vi "Apply Transfer Function.vi"() -> ()   [LabVIEW 2016]
uses:
  Globals/Motor Transfer.vi
panel:
  out "Left":T1
  out "Right":T1
  out "Right 2":cluster{dbl, "Right Value":dbl}[](graph)
  out "Left 2":cluster{dbl, "Left  Value":dbl}[](graph)
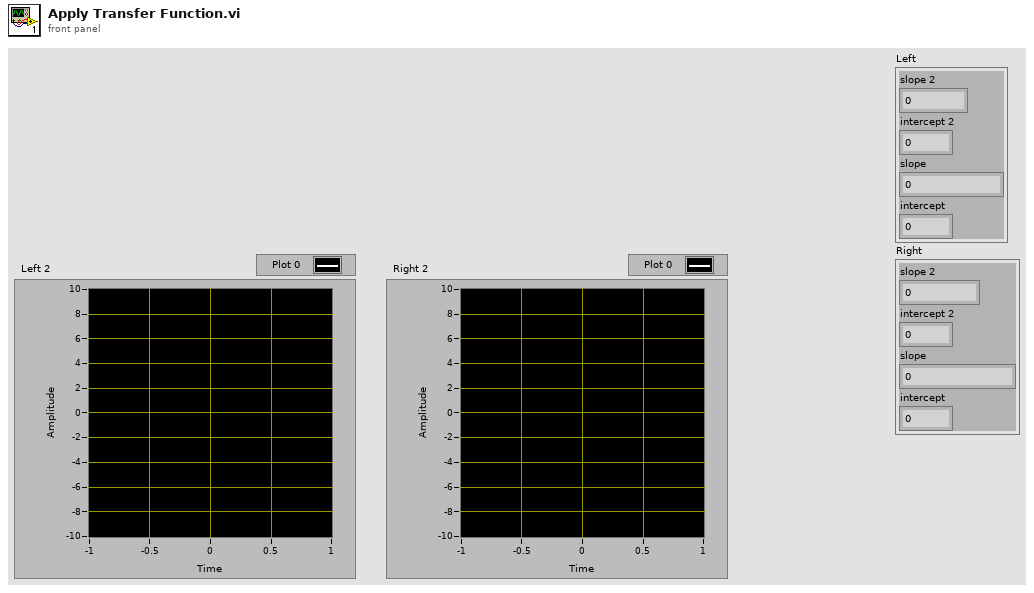
[diagram p1: front panel]
types:
  T1 = cluster{"slope 2":dbl, "intercept 2":dbl, "slope":dbl, "intercept":dbl}
  T2 = cluster{"p slope 2":dbl, "p intercept 2":dbl, "n slope":dbl, "n intercept":dbl}
  T3 = cluster{cluster{"p slope 2":dbl, "p intercept 2":dbl}, cluster{"n slope":dbl, "n intercept":dbl}}
  T4 = cluster{cluster{"p slope 2":dbl, "p intercept 2":dbl}, cluster{"n slope":dbl, "n intercept":dbl}}[]
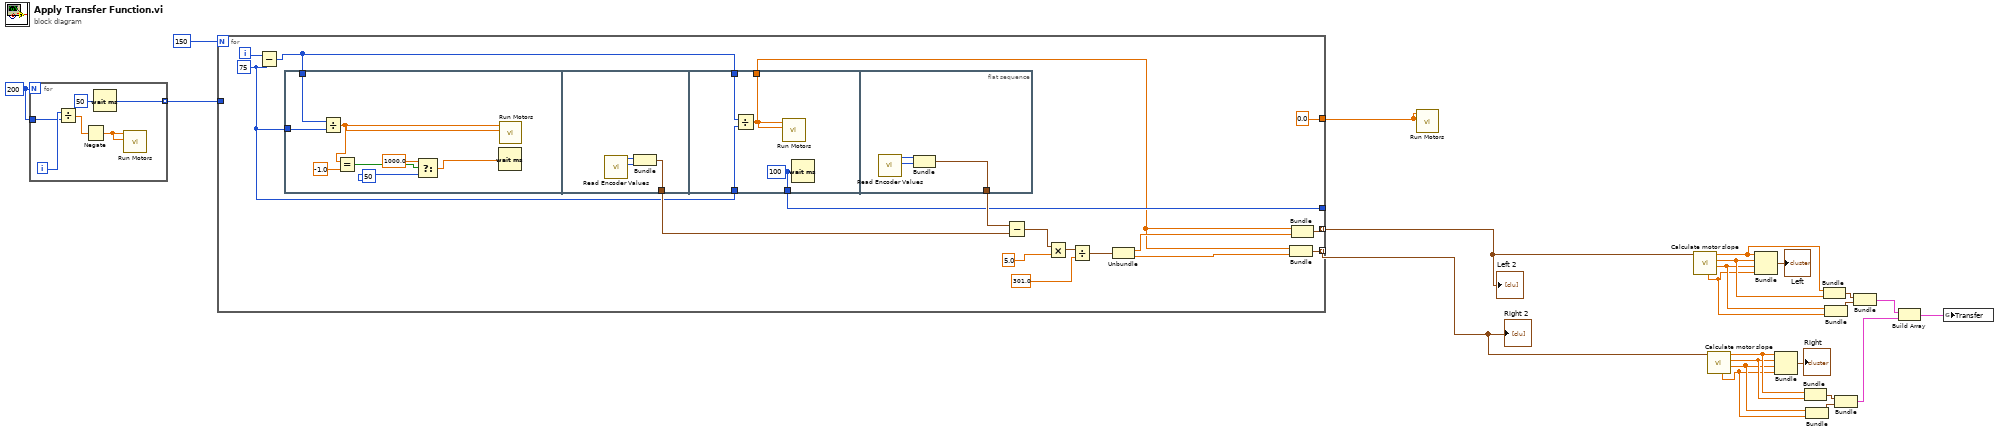
[diagram p0: block diagram]
diagram:
  w2 = 200
  n1 = for {
    N: w2 -> [_]
    tunnel: w2 -> [w27]
    tunnel: [w24] -> w1 mode=indexing
    i -> [w28]
    n2 = Divide(x=w28, y=w27) -> (x/y=w25:dbl)
    n3 = Negate(x=w25) -> (-x=w26:dbl)
    n4 = Wait (ms)(milliseconds to wait=u32 50) -> (millisecond timer value=w24:u32)
    n5 = call "Run Motors.vi"("Right motor side (-1..1)"=w26, "Left motor speed (-1..1)"=w26) -> ()  [unwired: 10 in]
  }
  n6 = for {
    N: 150 -> [_]
    tunnel: [w42] -> w21 mode=indexing
    tunnel: [w41] -> w20 mode=indexing
    tunnel: [0.0 ("Left motor speed (-1..1)")] -> w22
    tunnel: [w37] -> _
    tunnel: w1 -> [_]
    i -> [w39]
    w30 = 75 ("y")
    n7 = Subtract(x=w39, y=w30) -> (x-y=w38:i32)
    n8 = flat-sequence {
      tunnel: w38 -> [w54]
      tunnel: w30 -> [w47]
      tunnel: [w55] -> w45
      tunnel: w38 -> [w61]
      tunnel: [w60] -> w37
      tunnel: [w59] -> w36
      tunnel: w30 -> [w58]
      tunnel: [w62] -> w46
      frame #0 {
        n9 = Divide(x=w54, y=w47) -> (x/y=w53:dbl)
        n10 = Equal?(x=w53, y=-1.0) -> (x = y?=w51:bool)
        n11 = Select(t=1000.0, s=w51, f=u32 50 ("milliseconds to wait")) -> (s? t:f=w48:dbl)
        n12 = Wait (ms)(milliseconds to wait=w48) -> ()  [unwired: 1 out]
        n13 = call "Run Motors.vi"("Right motor side (-1..1)"=w53, "Left motor speed (-1..1)"=w53) -> ()  [unwired: 10 in]
      }
      frame #1 {
        n14 = call "Read Encoder Values.vi"() -> ("Right Value"=w56:i32, "Left  Value"=w57:i32)  [unwired: 10 in]
        n15 = Bundle("Left  Value"=w57, "Right Value"=w56) -> (w55:cluster{"Left  Value":i32, "Right Value":i32})  [unwired: 1 in]
      }
      frame #2 {
        w60 = u32 100 ("milliseconds to wait")
        n16 = Divide(x=w61, y=w58) -> (x/y=w59:dbl)
        n17 = call "Run Motors.vi"("Right motor side (-1..1)"=w59, "Left motor speed (-1..1)"=w59) -> ()  [unwired: 10 in]
        n18 = Wait (ms)(milliseconds to wait=w60) -> ()  [unwired: 1 out]
      }
      frame #3 {
        n19 = call "Read Encoder Values.vi"() -> ("Right Value"=w63:i32, "Left  Value"=w64:i32)  [unwired: 10 in]
        n20 = Bundle("Left  Value"=w64, "Right Value"=w63) -> (w62:cluster{"Left  Value":i32, "Right Value":i32})  [unwired: 1 in]
      }
    }
    n21 = Subtract(x=w46, y=w45) -> (x-y=w35:cluster{"Left  Value":i32, "Right Value":i32})
    n22 = Multiply(x=w35, y=5.0) -> (x*y=w33:cluster{"Left  Value":dbl, "Right Value":dbl})
    n23 = Divide(x=w33, y=301.0) -> (x/y=w31:cluster{"Left  Value":dbl, "Right Value":dbl})
    n24 = Unbundle(w31) -> ("Left  Value"=w44:dbl, "Right Value"=w43:dbl)
    n25 = Bundle(w36, "Right Value"=w43) -> (w41:cluster{dbl, "Right Value":dbl})  [unwired: 1 in]
    n26 = Bundle(w36, "Left  Value"=w44) -> (w42:cluster{dbl, "Left  Value":dbl})  [unwired: 1 in]
  }
  "Left 2" <- w21
  "Right 2" <- w20
  n27 = call "Run Motors.vi"("Right motor side (-1..1)"=w22, "Left motor speed (-1..1)"=w22) -> ()  [unwired: 10 in]
  n28 = call "Calculate motor slope.vi"("Array"=w21) -> ("n slope"=w11:dbl, "p intercept 2"=w12:dbl, "p slope 2"=w13:dbl, "n intercept"=w10:dbl)  [unwired: 7 in]
  n29 = call "Calculate motor slope.vi"("Array"=w20) -> ("n slope"=w4:dbl, "p intercept 2"=w5:dbl, "p slope 2"=w6:dbl, "n intercept"=w3:dbl)  [unwired: 7 in]
  n30 = Bundle("p slope 2"=w13, "p intercept 2"=w12, "n slope"=w11, "n intercept"=w10) -> (→"Left":T2)  [unwired: 1 in]
  n31 = Bundle("p slope 2"=w6, "p intercept 2"=w5, "n slope"=w4, "n intercept"=w3) -> (→"Right":T2)  [unwired: 1 in]
  n32 = Bundle("p slope 2"=w6, "p intercept 2"=w5) -> (w8:cluster{"p slope 2":dbl, "p intercept 2":dbl})  [unwired: 1 in]
  n33 = Bundle("n slope"=w4, "n intercept"=w3) -> (w9:cluster{"n slope":dbl, "n intercept":dbl})  [unwired: 1 in]
  n34 = Bundle("p slope 2"=w13, "p intercept 2"=w12) -> (w15:cluster{"p slope 2":dbl, "p intercept 2":dbl})  [unwired: 1 in]
  n35 = Bundle("n slope"=w11, "n intercept"=w10) -> (w14:cluster{"n slope":dbl, "n intercept":dbl})  [unwired: 1 in]
  n36 = Bundle(w8, w9) -> (w7:T3)  [unwired: 1 in]
  n37 = Bundle(w15, w14) -> (w16:T3)  [unwired: 1 in]
  n38 = Build Array(w16, w7) -> (w17:T4)
  n39 = global write "Motor Transfer.vi" "Transfer"(w17) -> ()
